vi "Collate_graphs.vi"(4 "R values":dbl[](array[numeric]), 5 "rho0":dbl[](array[numeric]), 6 "rho-":dbl[](array[numeric]), 7 "rho+":dbl[](array[numeric]), 8 "Gaussian SD in":dbl, 9 "AFP Range":cluster{"Numeric":i32, "Numeric 2":i32}, 10 "RF Range 2":cluster{"Numeric":i32, "Numeric 2":i32}, 11 "RF Range 1":cluster{"Numeric":i32, "Numeric 2":i32}) -> (2 "Q Graph":cluster{"Array":dbl[], "Array 2":dbl[]}, 3 "P Graph and Intensities and RF":cluster{"Array":dbl[], "Array":dbl[]}[](array[cluster]))   [LabVIEW 2018]
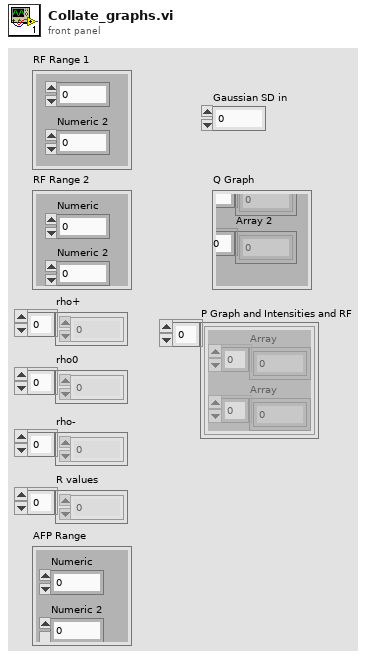
[diagram p1: front panel]
types:
  T1 = cluster{"R values":dbl[], "Output Array":dbl[]}[]
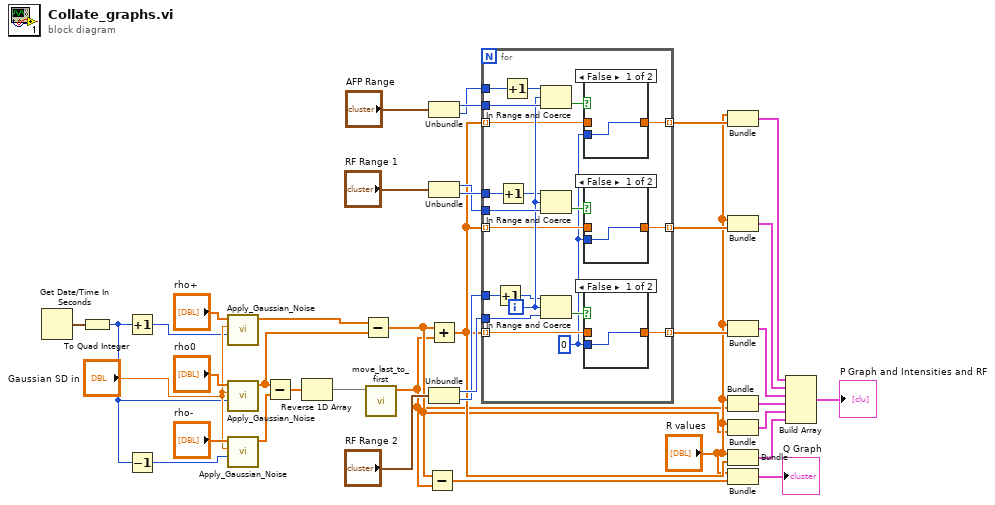
[diagram p0: block diagram]
diagram:
  n1 = Get Date/Time In Seconds() -> (seconds since 1Jan1904=w4:timestamp)
  n2 = To Quad Integer(1:w4) -> (0:w1:i64)
  n3 = Increment(x=w1) -> (x+1=w2:i64)
  n4 = Decrement(x=w1) -> (x-1=w3:i64)
  n5 = call "Apply_Gaussian_Noise.vi"("Seed in"=w2, "Gaussian SD in"="Gaussian SD in", "Array in"="rho+") -> ("Array out"=w8:dbl[])  [unwired: 8 in]
  n6 = call "Apply_Gaussian_Noise.vi"("Seed in"=w1, "Gaussian SD in"="Gaussian SD in", "Array in"="rho0") -> ("Array out"=w7:dbl[])  [unwired: 8 in]
  n7 = call "Apply_Gaussian_Noise.vi"("Seed in"=w3, "Gaussian SD in"="Gaussian SD in", "Array in"="rho-") -> ("Array out"=w6:dbl[])  [unwired: 8 in]
  n8 = Subtract(x=w7, y=w6) -> (x-y=w35:dbl[])
  n9 = Reverse 1D Array(array=w35) -> (reversed array=w10:dbl[])
  n10 = Subtract(x=w8, y=w7) -> (x-y=w13:dbl[])
  n11 = call "move_last_to_first.vi"("Input array"=w10) -> ("Output Array"=w9:dbl[])  [unwired: 10 in]
  n12 = Subtract(x=w13, y=w9) -> (x-y=w21:dbl[])
  n13 = Unbundle("AFP Range") -> ("Numeric"=w27:i32, "Numeric 2"=w26:i32)
  n14 = Unbundle("RF Range 1") -> ("Numeric"=w30:i32, "Numeric 2"=w31:i32)
  n15 = Add(x=w13, y=w9) -> (x+y=w22:dbl[])
  n16 = Unbundle("RF Range 2") -> ("Numeric"=w29:i32, "Numeric 2"=w28:i32)
  n17 = for {
    tunnel: w31 -> [w58]
    tunnel: w30 -> [w57]
    tunnel: w29 -> [w53]
    tunnel: w28 -> [w52]
    tunnel: w27 -> [w51]
    tunnel: w26 -> [w50]
    tunnel: w22 -> [w48] mode=indexing
    tunnel: w22 -> [w47] mode=indexing
    tunnel: w22 -> [w46] mode=indexing
    tunnel: [w45] -> w25 mode=indexing
    tunnel: [w44] -> w23 mode=indexing
    tunnel: [w43] -> w24 mode=indexing
    i -> [w49]
    w42 = 0
    n18 = Increment(x=w52) -> (x+1=w41:i32)
    n19 = Increment(x=w58) -> (x+1=w40:i32)
    n20 = Increment(x=w50) -> (x+1=w39:i32)
    n21 = In Range and Coerce(upper limit=w39, x=w49, lower limit=w51) -> (In Range?=w56:bool)  [unwired: 1 out]
    n22 = In Range and Coerce(upper limit=w40, x=w49, lower limit=w57) -> (In Range?=w54:bool)  [unwired: 1 out]
    n23 = In Range and Coerce(upper limit=w41, x=w49, lower limit=w53) -> (In Range?=w55:bool)  [unwired: 1 out]
    n24 = case shown="False" w56 {
      tunnel: w46 -> [_ w60]
      tunnel: [w59 w60] -> w43
      tunnel: w42 -> [w59 _]
      frame False {
      }
      frame True {
      }
    }
    n25 = case shown="False" w54 {
      tunnel: w48 -> [_ w64]
      tunnel: [w63 w64] -> w45
      tunnel: w42 -> [w63 _]
      frame False {
      }
      frame True {
      }
    }
    n26 = case shown="False" w55 {
      tunnel: w47 -> [_ w62]
      tunnel: [w61 w62] -> w44
      tunnel: w42 -> [w61 _]
      frame False {
      }
      frame True {
      }
    }
  }
  n27 = Bundle("R values"="R values", w24) -> (w16:cluster{"R values":dbl[], dbl[]})  [unwired: 1 in]
  n28 = Bundle("R values"="R values", w25) -> (w20:cluster{"R values":dbl[], dbl[]})  [unwired: 1 in]
  n29 = Bundle("R values"="R values", w23) -> (w19:cluster{"R values":dbl[], dbl[]})  [unwired: 1 in]
  n30 = Bundle("R values"="R values", "Output Array"=w9) -> (w11:cluster{"R values":dbl[], "Output Array":dbl[]})  [unwired: 1 in]
  n31 = Bundle("R values"="R values", w13) -> (w12:cluster{"R values":dbl[], dbl[]})  [unwired: 1 in]
  n32 = Bundle("R values"="R values", w22) -> (w15:cluster{"R values":dbl[], dbl[]})  [unwired: 1 in]
  n33 = Bundle("R values"="R values", w21) -> (→"Q Graph":cluster{"R values":dbl[], dbl[]})  [unwired: 1 in]
  n34 = Build Array(w16, w20, w19, w11, w12, w15) -> (→"P Graph and Intensities and RF":T1)
